vi "Result_Test.vi"(8 "error in (no error)":errorcluster caption="entrée d'erreur (pas d'erreur)", 11 "Get_Voltage en entrée":refnum<class "Nodon_Get_Product_ID.lvclass">) -> (0 "error out":errorcluster caption="sortie d'erreur", 3 "Get_Voltage en sortie":refnum<class "Nodon_Get_Product_ID.lvclass">)   [LabVIEW 2020, in "Library Test.lvlib" / "Nodon_Get_Product_ID.lvclass"]
uses:
  Nodon_Get_Product_ID.lvclass
  C:/Users/ngarcin/OneDrive - Altyor/Standard TB/Suite TB45/Class/Test/Test (Default)/Test (Default).lvclass
  Commun VI/TypeDef/Variable Printable.ctl
  JSON API/JSON Value/Set from JSON string.vi
  JSON API/JSON Value/JSON Value.lvclass
  Nodon_Send_Command_UART.lvclass
  JSON API/Variant JSON/Variant JSON.lvlib
  JSON API/Get Polymorphic/JSON GetSet.lvlib
  Commun VI/Library Commun.lvlib
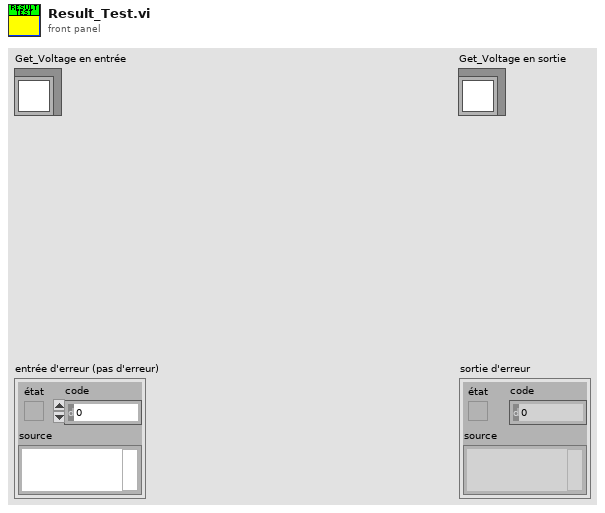
[diagram p1: front panel]
types:
  T1 = typedef "Variable Printable.ctl" = string
  T2 = enum16{"Get Variable", "Get All Variables", "Set Variable", "Delete Variable", "Delete All Variable"}
  T3 = cluster{"Commande Type":string, "Command ID":string, "Data":string, "Error":string}
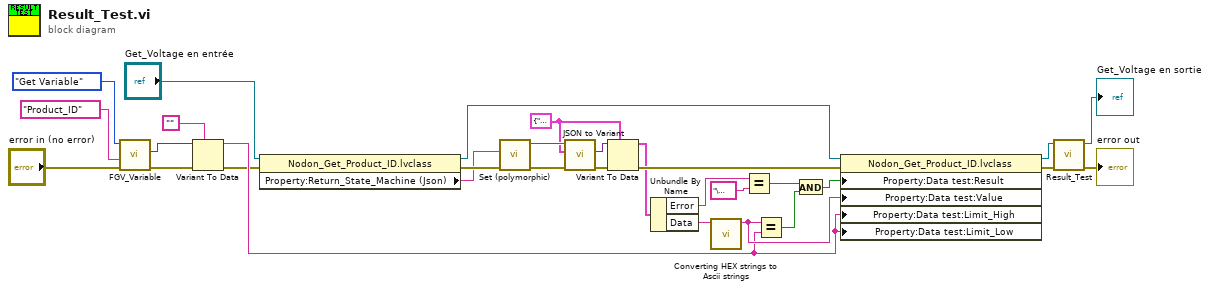
[diagram p0: block diagram]
diagram:
  w17 = T3 {"Commande Type"="", "Command ID"="", "Data"="", "Error"=""}
  n1 = call "FGV_Variable.vi"("error in (no error)"="error in (no error)", "Variable"=T1 "Product_ID", "Function"=T2."Get Variable") -> ("error out"=w10:errorcluster, "Data Out"=w9:variant)  [unwired: 6 in, 1 out]
  n2 = Variant To Data(error in=w10, type="", Variant=w9) -> (data=w2:string, error out=w1:errorcluster)
  n3 = property class="Nodon_Get_Product_ID.lvclass"(reference="Get_Voltage en entrée", error in=w1) -> (reference out=w28:refnum<class "Nodon_Get_Product_ID.lvclass">, error out=w23:errorcluster, "Property:Return_State_Machine (Json)"=w21:string)
  n4 = call-poly "Set (polymorphic).vi"("error in (no error)"=w23, "JSON stream"=w21) -> ("error out"=w25:errorcluster, "JSON Value out"=w27:refnum<class "JSON Value.lvclass">)  [unwired: 7 in, 1 out]
  n5 = call "JSON to Variant.vi"("error in (no error)"=w25, "Variant (Data Type)"=w17, "JSON Value"=w27) -> ("error out"=w26:errorcluster, "Variant out"=w24:variant)  [unwired: 7 in]
  n6 = Variant To Data(error in=w26, type=w17, Variant=w24) -> (data=w20:T3, error out=w22:errorcluster)
  n7 = Unbundle By Name(w20) -> ("Error"=w19:string, "Data"=w13:string)
  n8 = call "Converting HEX strings to Ascii strings.vi"("chaîne IN"=w13) -> ("Chaîne OUT"=w6:string)  [unwired: 9 in, 1 out]
  n9 = Equal?(x=w19, y="\u0000") -> (x = y?=w4:bool)
  n10 = Equal?(x=w6, y=w2) -> (x = y?=w5:bool)
  n11 = And(x=w4, y=w5) -> (x .and. y?=w3:bool)
  n12 = property class="Nodon_Get_Product_ID.lvclass"(reference=w28, error in=w22, "Property:Data test:Result"=w3, "Property:Data test:Value"=w6, "Property:Data test:Limit_High"=w2, "Property:Data test:Limit_Low"=w2) -> (reference out=w15:refnum<class "Nodon_Get_Product_ID.lvclass">, error out=w14:errorcluster)
  n13 = call-parent "Result_Test.vi"("error in (no error)"=w14, "Get_Voltage en entrée"=w15) -> ("error out"=→"error out":errorcluster, "Get_Voltage en sortie"=→"Get_Voltage en sortie":refnum<class "Nodon_Get_Product_ID.lvclass">)  [unwired: 8 in]
